vi "XW_Create_Map_tf_old.vi"() -> ()   [LabVIEW 2011]
uses:
  Controls/File_Selector_Type.ctl
  Controls/Cal_Inst_type.ctl
panel:
  out "2D data array 2":dbl[][](array[numeric])
  out "index of element":i32
  in  "At Dialog Prompt Post Process":T1
  out "String":string
  out "2D data array":dbl[][](array[numeric]) format="%.2f"
  out "Off 2":dbl
  out "Gain 2":dbl
  out "Off 1":dbl
  out "Gain 1":dbl
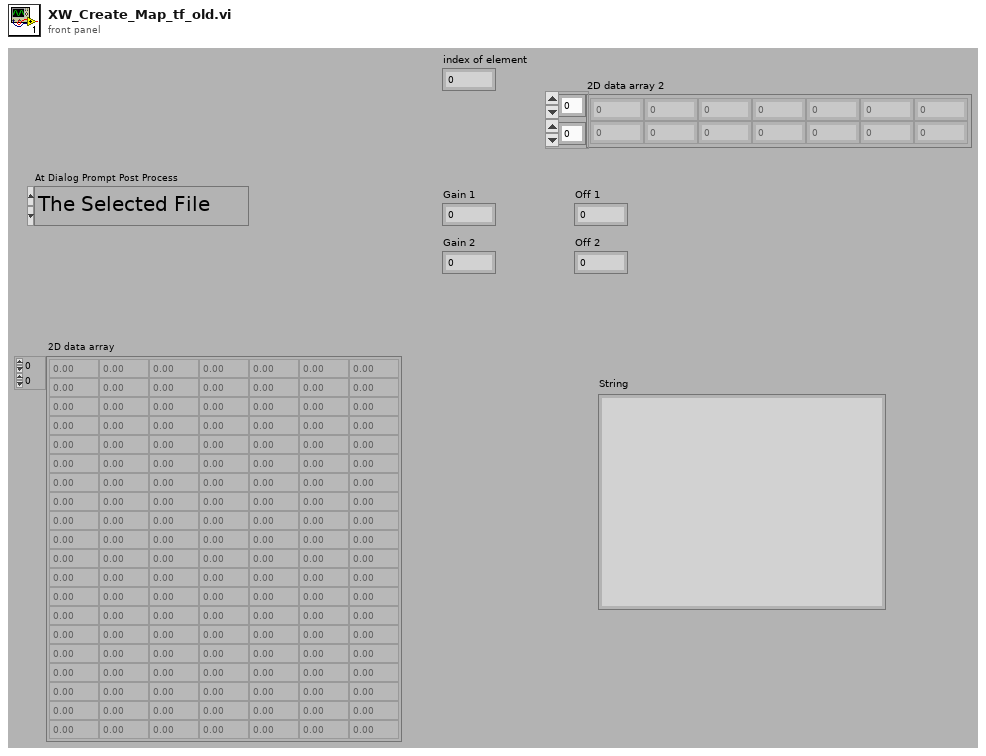
[diagram p1: front panel]
types:
  T1 = typedef "File_Selector_Type.ctl" = enum16{"The Selected File", "The Selected Folder", "Files containing the search string in the selected folder", "All files listed in selected file"}
  T2 = typedef "Cal_Inst_type.ctl" = enum16{"Propeller anemometer", "Pressure Transducer", "Hot wire", "Cross wire velocity", "Cross wire angle", "Generic Linear", "Generic Polynomial", "Generic BackPoly", "Fast FID", "Thermocouple", "Cold wire", "Pulsed Wire"}
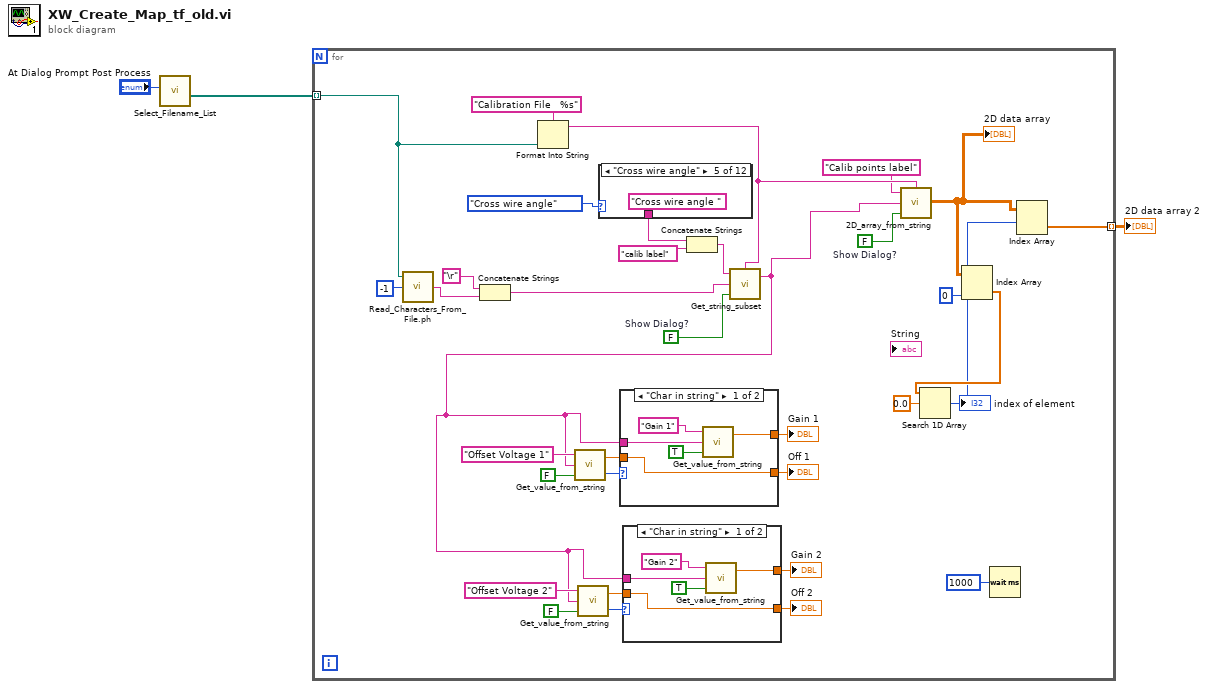
[diagram p0: block diagram]
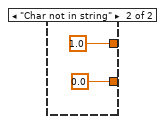
[diagram p2: hidden frame]
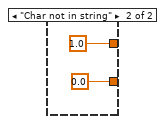
[diagram p3: hidden frame]
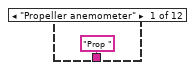
[diagram p4: hidden frame]
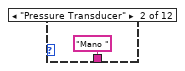
[diagram p5: hidden frame]
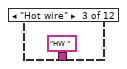
[diagram p6: hidden frame]
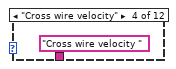
[diagram p7: hidden frame]
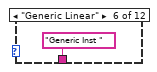
[diagram p8: hidden frame]
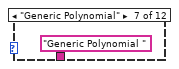
[diagram p9: hidden frame]
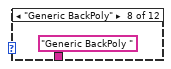
[diagram p10: hidden frame]
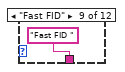
[diagram p11: hidden frame]
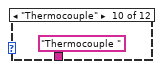
[diagram p12: hidden frame]
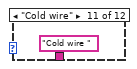
[diagram p13: hidden frame]
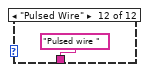
[diagram p14: hidden frame]
diagram:
  n1 = call "Select_Filename_List.vi"("At Dialog Prompt Post Process"="At Dialog Prompt Post Process") -> ("Selected files"=w3:path[])  [unwired: 5 in, 2 out]
  n2 = for {
    tunnel: w3 -> [w12] mode=indexing
    tunnel: [w4] -> w1 mode=indexing
    w27 = FALSE  # Show Dialog?
    w35 = FALSE  # Show Dialog?
    n3 = call "Read_Characters_From_File.ph.vi"("file path (dialog if empty)"=w12, "number of characters (all:-1)"=-1) -> ("character string"=w37:string)  [unwired: 7 out]
    n4 = Concatenate Strings("\r", w37) -> (w17:string)
    n5 = Format Into String(format string="Calibration File   %s", w12) -> (resulting string=w29:string)  [unwired: 2 in, 1 out]
    n6 = case shown="\"Cross wire angle\"" Cal_Inst_type."Cross wire angle" ("Instrument type") {
      tunnel: ["Prop " "Mano " "HW " "Cross wire velocity " "Cross wire angle " "Generic Inst " "Generic Polynomial " "Generic BackPoly " "Fast FID " "Thermocouple " "Cold wire " "Pulsed wire "] -> w34
      frame "Propeller anemometer" {
      }
      frame "Pressure Transducer" {
      }
      frame "Hot wire" {
      }
      frame "Cross wire velocity" {
      }
      frame "Cross wire angle" {
      }
      frame "Generic Linear" {
      }
      frame "Generic Polynomial" {
      }
      frame "Generic BackPoly" {
      }
      frame "Fast FID" {
      }
      frame "Thermocouple" {
      }
      frame "Cold wire" {
      }
      frame "Pulsed Wire" {
      }
    }
    n7 = Concatenate Strings(w34, "calib label") -> (w33:string)
    n8 = call "Get_string_subset.vi"("String Name"=w29, "Show Dialog?"=w35, "String to split"=w17, "File Label"=w33) -> ("Output string"=w10:string)  [unwired: 1 out]
    n9 = call "Get_value_from_string.vi"("Show Dialog?"=FALSE, "Input string"=w10, "Variable name"="Offset Voltage 1") -> ("Status"=w23:enum16{"Char in string", "Char not in string"}, "Value"=w22:dbl)
    n10 = call "Get_value_from_string.vi"("Show Dialog?"=FALSE, "Input string"=w10, "Variable name"="Offset Voltage 2") -> ("Status"=w20:enum16{"Char in string", "Char not in string"}, "Value"=w21:dbl)
    n11 = case shown="\"Char in string\"" w23 {
      tunnel: w10 -> [w49 _]
      tunnel: [w46 1.0 ("Value")] -> w16
      tunnel: w22 -> [w45 _]
      tunnel: [w45 0.0 ("Value")] -> w15
      frame "Char in string" {
        n12 = call "Get_value_from_string.vi"("Show Dialog?"=TRUE, "Input string"=w49, "Variable name"="Gain 1") -> ("Value"=w46:dbl)  [unwired: 1 out]
      }
      frame "Char not in string" {
      }
    }
    "Gain 1" <- w16
    "Off 1" <- w15
    n13 = case shown="\"Char in string\"" w20 {
      tunnel: w10 -> [w42 _]
      tunnel: [w39 1.0 ("Value")] -> w14
      tunnel: w21 -> [w38 _]
      tunnel: [w38 0.0 ("Value")] -> w13
      frame "Char in string" {
        n14 = call "Get_value_from_string.vi"("Show Dialog?"=TRUE, "Input string"=w42, "Variable name"="Gain 2") -> ("Value"=w39:dbl)  [unwired: 1 out]
      }
      frame "Char not in string" {
      }
    }
    "Gain 2" <- w14
    "Off 2" <- w13
    n15 = call "2D_array_from_string.vi"("String Name"=w29, "Show Dialog?"=w27, "Input string"=w10, "Array title"="Calib points label") -> ("2D data array"=w5:dbl[][])
    "2D data array" <- w5
    n16 = Index Array(array=w5, index (col)=0 ("disabled index (col)")) -> (element=w7:dbl[])  [unwired: 1 in]
    n17 = Search 1D Array(1D array=w7, element=0.0) -> (index of element=w6:i32)  [unwired: 1 in]
    "index of element" <- w6
    n18 = Wait (ms)(milliseconds to wait=u32 1000) -> ()  [unwired: 1 out]
    n19 = Index Array(array=w5, index (row)=w6) -> (element=w4:dbl[])  [unwired: 1 in]
  }
  "2D data array 2" <- w1
